vi "VariableWriteUI.vi"(10 "VariableFill":refnum<class "Variable.lvclass">, 11 "VariableManagerRef in":refnum<vi>) -> (2 "VariableWrote":refnum<class "Variable.lvclass">, 3 "VariableManagerRef out":refnum<vi>)   [LabVIEW 2013]
doc: "Create a window for add/edit variable of the given VariableManager reference. VariableWrote is returned when the user successfully add/edit the variable. VariableWrote has empty name if the user cancel the operation.\n\nThe name of VariableFill will determine the operation. \nIf the name of VariableFill already exists, the operation is editing the variable.\nIf the name of VariableFill does not exists, the operation is adding a variable."
uses:
  Variable/Variable.lvclass
  VariableManager/VariableManager.lvclass
  API/VariableManagerAPI.lvlib
panel:
  out "Operation":string
  in  "OK Button":bool
  in  "Cancel Button":bool
  in  "InformIgor":bool caption="Inform Igor?"
  in  "Sequence":bool caption="Sequence?"
  in  "SequenceFunction":string caption="Sequence Function"
  in  "DefaultValue":dbl caption="Default Value" format="%#_15p"
  in  "VariableName":string caption="Variable Name"
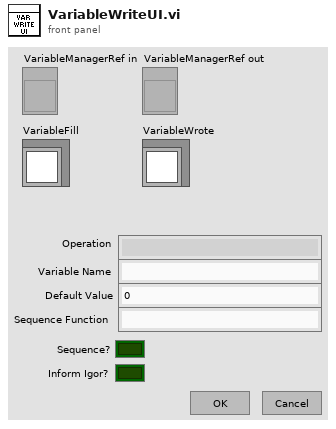
[diagram p1: front panel]
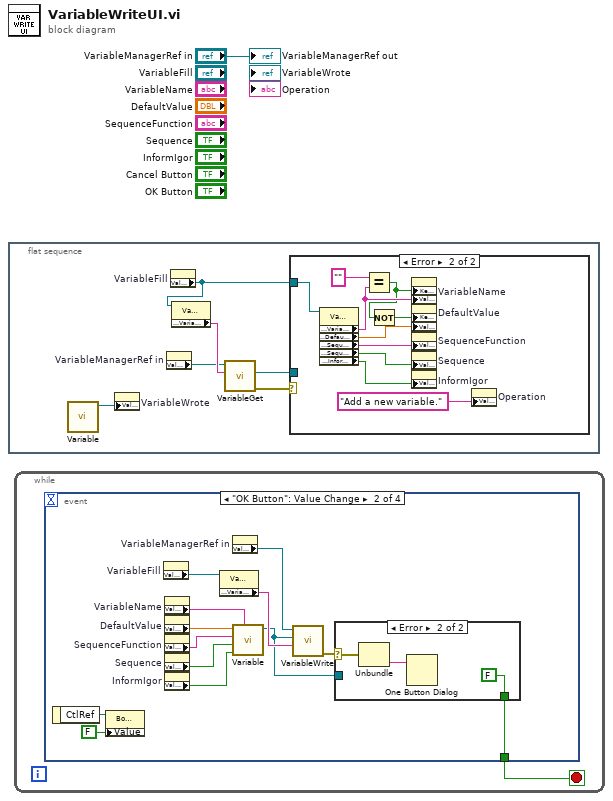
[diagram p0: block diagram]
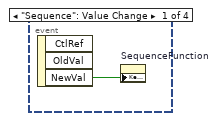
[diagram p2: hidden frame]
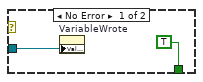
[diagram p3: hidden frame]
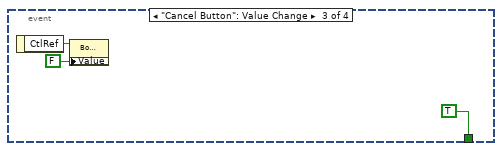
[diagram p4: hidden frame]
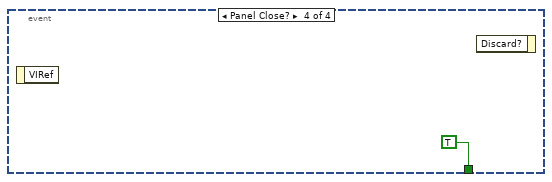
[diagram p5: hidden frame]
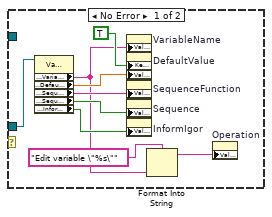
[diagram p6: hidden frame]
diagram:
  n1 = flat-sequence {
    frame #0 {
      n2 = call "Variable.vi"() -> ("Variable"=w2:refnum<class "Variable.lvclass">)  [unwired: 11 in]
      n3 = property on="VariableWrote" class="LVClassControl (strict)"("Value"=w2) -> ()  [unwired: 2 in, 2 out]
      n4 = property on="VariableManagerRef in" class="LVObjRef (strict)"() -> ("Value"=w6:refnum<vi>)  [unwired: 2 in, 2 out]
      n5 = property on="VariableFill" class="LVClassControl (strict)"() -> ("Value"=w3:refnum<class "Variable.lvclass">)  [unwired: 2 in, 2 out]
      n6 = property class="Variable.lvclass"(reference=w3) -> ("Accessors:VariableName"=w7:string)  [unwired: 1 in, 2 out]
      n7 = call "VariableGet.vi"("VariableName"=w7, "VariableManagerRef in"=w6) -> ("error out"=w5:errorcluster, "Variable"=w4:refnum<class "Variable.lvclass">)  [unwired: 7 in, 1 out]
      n8 = case shown="Error" w5 {
        tunnel: w4 -> [w11 _]
        tunnel: w3 -> [_ w22]
        frame No Error {
          n9 = property class="Variable.lvclass"(reference=w11) -> ("Accessors:VariableName"=w9:string, "Accessors:DefaultValue"=w16:dbl, "Accessors:SequenceFunction"=w15:string, "Accessors:Sequence"=w14:bool, "Accessors:InformIgor"=w13:bool)  [unwired: 1 in, 2 out]
          n10 = property on="VariableName" class="Str"("Value"=w9) -> ()  [unwired: 2 in, 2 out]
          n11 = property on="DefaultValue" class="DigNum (strict)"("Key Focus"=TRUE, "Value"=w16) -> ()  [unwired: 2 in, 2 out]
          n12 = property on="SequenceFunction" class="Str"("Value"=w15) -> ()  [unwired: 2 in, 2 out]
          n13 = property on="Sequence" class="Bool (strict)"("Value"=w14) -> ()  [unwired: 2 in, 2 out]
          n14 = property on="InformIgor" class="Bool (strict)"("Value"=w13) -> ()  [unwired: 2 in, 2 out]
          n15 = Format Into String(format string="Edit variable \"%s\"", w9) -> (resulting string=w8:string)  [unwired: 2 in, 1 out]
          n16 = property on="Operation" class="Str"("Value"=w8) -> ()  [unwired: 2 in, 2 out]
        }
        frame Error {
          n17 = property class="Variable.lvclass"(reference=w22) -> ("Accessors:VariableName"=w20:string, "Accessors:DefaultValue"=w26:dbl, "Accessors:SequenceFunction"=w25:string, "Accessors:Sequence"=w24:bool, "Accessors:InformIgor"=w23:bool)  [unwired: 1 in, 2 out]
          n18 = Equal?(x="", y=w20) -> (x = y?=w18:bool)
          n19 = Not(x=w18) -> (.not. x?=w17:bool)
          n20 = property on="VariableName" class="Str"("Key Focus"=w18, "Value"=w20) -> ()  [unwired: 2 in, 2 out]
          n21 = property on="DefaultValue" class="DigNum (strict)"("Key Focus"=w17, "Value"=w26) -> ()  [unwired: 2 in, 2 out]
          n22 = property on="SequenceFunction" class="Str"("Value"=w25) -> ()  [unwired: 2 in, 2 out]
          n23 = property on="Sequence" class="Bool (strict)"("Value"=w24) -> ()  [unwired: 2 in, 2 out]
          n24 = property on="InformIgor" class="Bool (strict)"("Value"=w23) -> ()  [unwired: 2 in, 2 out]
          n25 = property on="Operation" class="Str"("Value"="Add a new variable.") -> ()  [unwired: 2 in, 2 out]
        }
      }
    }
  }
  n26 = while {
    stop <- w27 stop-if-true
    n27 = event shown="[1] \"OK Button\": Value Change" {
      selector: _ -> [_ _ _ _]
      dyn-events: _ -> [_ _ _ _]
      timeout: _ -> [_ _ _ _]
      tunnel: [_ w30 TRUE TRUE] -> w27
      event "Sequence": Value Change {
        n28 = event-data() -> ("NewVal"=w28:bool)  [unwired: 1 in, 2 out]
        n29 = property on="SequenceFunction" class="Str"("Key Focus"=w28) -> ()  [unwired: 2 in, 2 out]
      }
      event "OK Button": Value Change {
        n30 = event-data() -> ("CtlRef"=w41:refnum<vi>)  [unwired: 1 in]
        n31 = property class="Bool (strict)"(reference=w41, "Value"=FALSE) -> ()  [unwired: 1 in, 2 out]
        n32 = property on="VariableFill" class="LVClassControl (strict)"() -> ("Value"=w34:refnum<class "Variable.lvclass">)  [unwired: 2 in, 2 out]
        n33 = property on="VariableName" class="Str"() -> ("Value"=w39:string)  [unwired: 2 in, 2 out]
        n34 = property on="DefaultValue" class="DigNum (strict)"() -> ("Value"=w38:dbl)  [unwired: 2 in, 2 out]
        n35 = property on="SequenceFunction" class="Str"() -> ("Value"=w37:string)  [unwired: 2 in, 2 out]
        n36 = property on="Sequence" class="Bool (strict)"() -> ("Value"=w36:bool)  [unwired: 2 in, 2 out]
        n37 = property on="InformIgor" class="Bool (strict)"() -> ("Value"=w35:bool)  [unwired: 2 in, 2 out]
        n38 = property class="Variable.lvclass"(reference=w34) -> ("Accessors:VariableName"=w32:string)  [unwired: 1 in, 2 out]
        n39 = property on="VariableManagerRef in" class="LVObjRef (strict)"() -> ("Value"=w33:refnum<vi>)  [unwired: 2 in, 2 out]
        n40 = call "Variable.vi"("VariableName"=w39, "InformIgor"=w35, "Sequence"=w36, "SequenceFunction"=w37, "DefaultValue"=w38) -> ("Variable"=w29:refnum<class "Variable.lvclass">)  [unwired: 6 in]
        n41 = call "VariableWrite.vi"("OriginalName"=w32, "Variable"=w29, "VariableManagerRef in"=w33) -> ("error out"=w31:errorcluster)  [unwired: 7 in, 1 out]
        n42 = case shown="Error" w31 {
          selector: w31 -> [_ w45]
          tunnel: [TRUE FALSE] -> w30
          tunnel: w29 -> [w42 _]
          frame No Error {
            n43 = property on="VariableWrote" class="LVClassControl (strict)"("Value"=w42) -> ()  [unwired: 2 in, 2 out]
          }
          frame Error {
            n44 = Unbundle(w45) -> ("source"=w44:string)  [unwired: 2 out]
            n45 = One Button Dialog(message=w44) -> ()  [unwired: 1 in, 1 out]
          }
        }
      }
      event "Cancel Button": Value Change {
        n46 = event-data() -> ("CtlRef"=w48:refnum<vi>)  [unwired: 1 in]
        n47 = property class="Bool (strict)"(reference=w48, "Value"=FALSE) -> ()  [unwired: 1 in, 2 out]
      }
      event Panel Close? {
        n48 = event-data() -> ()  [unwired: 1 in, 1 out]
        n49 = event-data() -> ()  [unwired: 2 in, 1 out]
      }
    }
  }
  "VariableManagerRef out" <- "VariableManagerRef in"
